vi "complex-to-xy-plot.vi"(10 "complex-vector":cdb[](array[numeric]), 11 "number-of-points":i32) -> (3 "xy-plot-output":cluster{dbl[], dbl[]}[](array[cluster]))   [LabVIEW 2024]
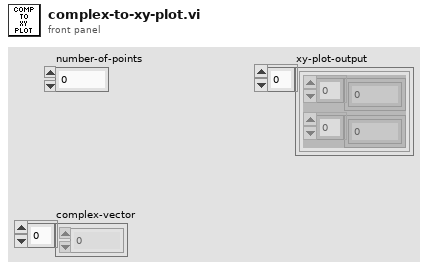
[diagram p1: front panel]
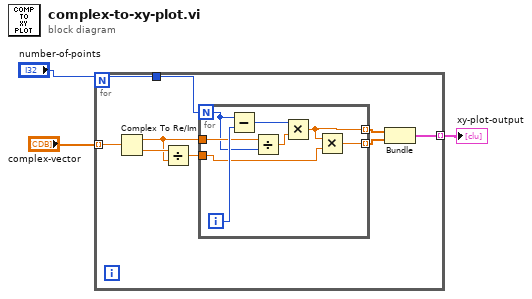
[diagram p0: block diagram]
diagram:
  n1 = for {
    tunnel: [w5] -> w2 mode=indexing
    tunnel: "complex-vector" -> [w8] mode=indexing
    tunnel: "number-of-points" -> [w4]
    n2 = Complex To Re/Im(x + iy=w8) -> (x=w9:dbl, y=w11:dbl)
    n3 = Divide(x=w11, y=w9) -> (x/y=w10:dbl)
    n4 = for {
      N: w4 -> [w17]
      tunnel: w10 -> [w14]
      tunnel: w9 -> [w18]
      tunnel: [w13] -> w7 mode=indexing
      tunnel: [w12] -> w6 mode=indexing
      i -> [w19]
      n5 = Subtract(x=w17, y=w19) -> (x-y=w16:i32)
      n6 = Divide(x=w18, y=w17) -> (x/y=w15:dbl)
      n7 = Multiply(x=w16, y=w15) -> (x*y=w13:dbl)
      n8 = Multiply(x=w13, y=w14) -> (x*y=w12:dbl)
    }
    n9 = Bundle(w7, w6) -> (w5:cluster{dbl[], dbl[]})  [unwired: 1 in]
  }
  "xy-plot-output" <- w2
